vi "GoBirdBath - Test.vi"() -> ()   [LabVIEW 2017]
panel:
  out "error out":errorcluster
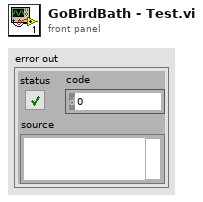
[diagram p1: front panel]
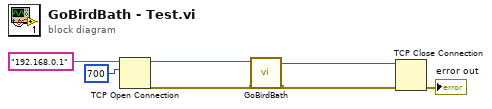
[diagram p0: block diagram]
diagram:
  n1 = TCP Open Connection(address="192.168.0.1", remote port or service name=u16 700) -> (connection ID=w4:refnum<k5>, error out=w3:errorcluster)  [unwired: 3 in]
  n2 = call "GoBirdBath.vi"("error in (no error)"=w3, "TCP Network Connection in"=w4) -> ("error out"=w1:errorcluster, "TCP Network Connection out"=w2:refnum<k5>)  [unwired: 6 in, 2 out]
  n3 = TCP Close Connection(connection ID=w2, error in (no error)=w1) -> (error out=→"error out":errorcluster)  [unwired: 1 in, 1 out]
